vi "File check 2.0.vi"(8 "error in (no error)":errorcluster, 9 "reference":refnum<vi>, 10 "Numeric":i32, 11 "path":path) -> (0 "error out":errorcluster, 3 "Next State":string)   [LabVIEW 2016]
uses:
  Type Defs/File Check 2.0 control.ctl
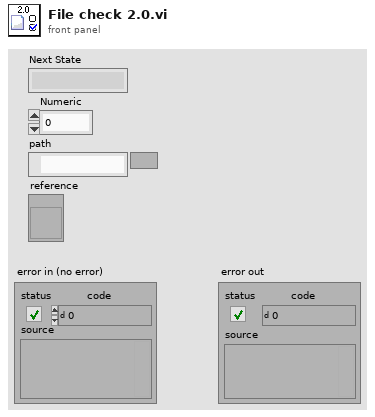
[diagram p1: front panel]
types:
  T1 = typedef "File Check 2.0 control.ctl" = enum16{"File Check", "Secondary check", "Refresh Google Drive"}
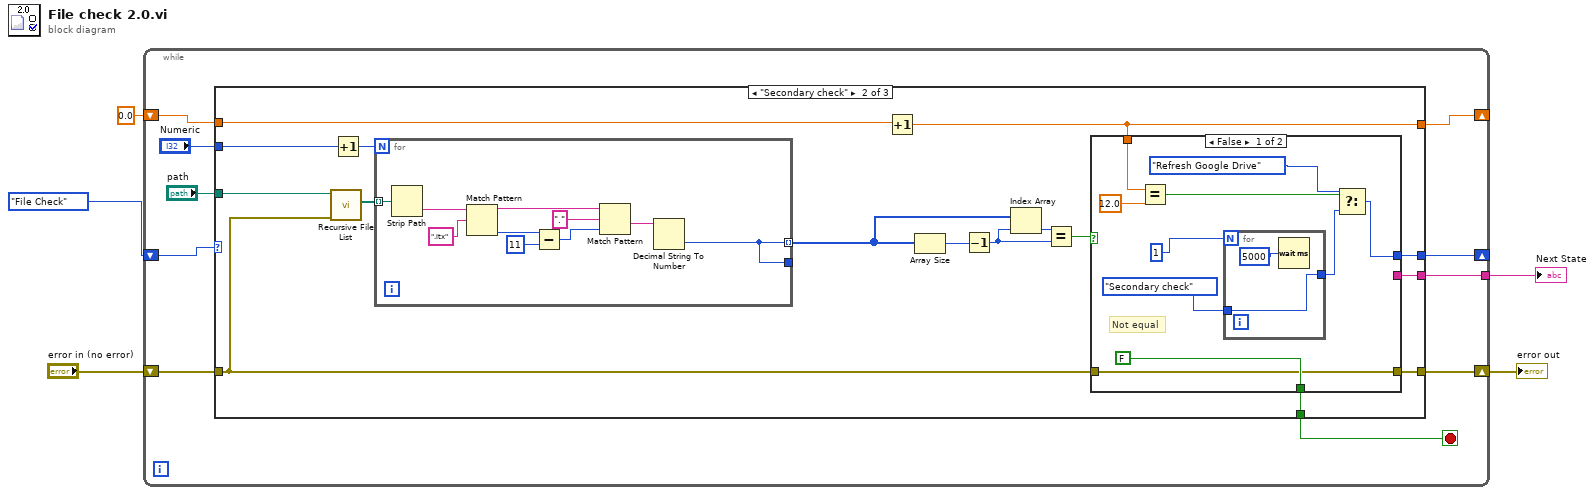
[diagram p0: block diagram]
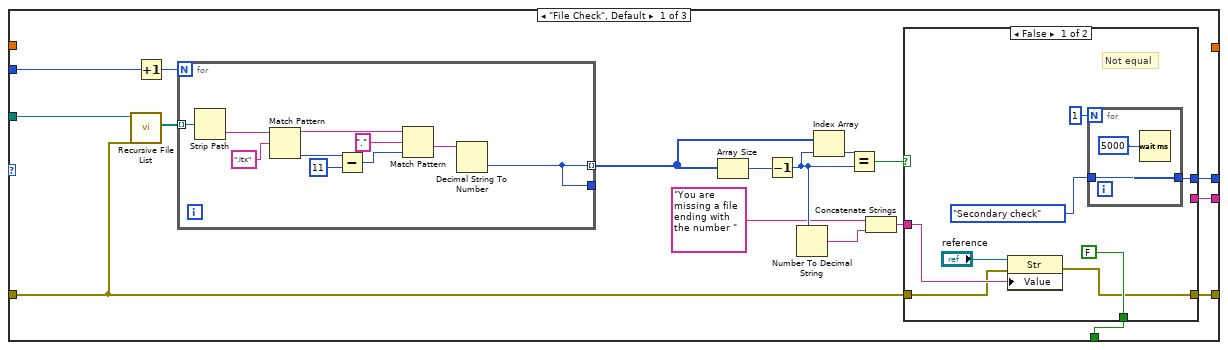
[diagram p2: hidden frame]
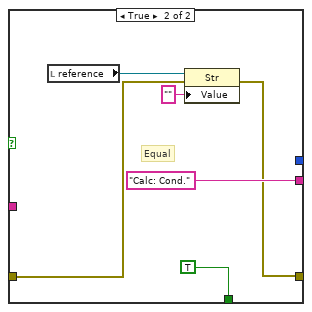
[diagram p3: hidden frame]
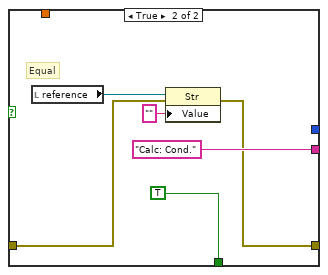
[diagram p4: hidden frame]
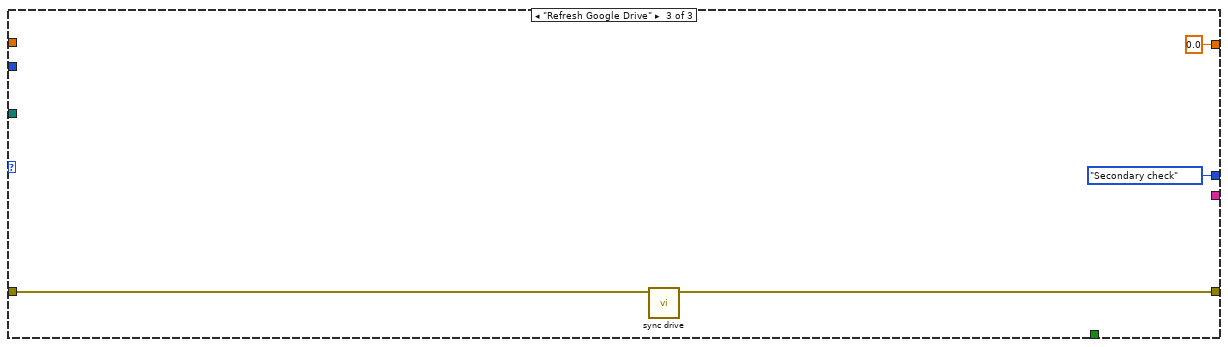
[diagram p5: hidden frame]
diagram:
  n1 = while {
    tunnel: [w15] -> w5
    shift-right: [w12] -> _
    shift-left: File_Check_2.0_control."File Check" -> [w11]
    shift-right: [w10] -> w2
    shift-left: "error in (no error)" -> [w7]
    shift-right: [w8] -> _
    shift-left: 0.0 -> [w9]
    stop <- w6 stop-if-true
    n2 = case shown="\"Secondary check\"" w11 {
      tunnel: [w25 w67 _] -> w15
      tunnel: [w23 w66 _] -> w6
      tunnel: "Numeric" -> [w26 w65 _]
      tunnel: "path" -> [w18 w63 _]
      tunnel: [w24 w64 File_Check_2.0_control."Secondary check"] -> w12
      tunnel: [w16 w62 w103] -> w10
      tunnel: w9 -> [_ w61 _]
      tunnel: [_ w60 0.0] -> w8
      tunnel: w7 -> [w17 w59 w104]
      frame "File Check", Default {
        n3 = call <vilib>:"Recursive File List.vi"("error in (no error)"=w17, "Folder Path"=w18) -> ("All Files in Dir"=w32:path[])  [unwired: 6 in, 3 out]
        n4 = Increment(x=w26) -> (x+1=w27:i32)
        n5 = for {
          N: w27 -> [_]
          tunnel: [w49] -> w28 mode=indexing
          tunnel: w32 -> [w50] mode=indexing
          tunnel: [w49] -> _
          n6 = Strip Path(path=w50) -> (name=w58:string)  [unwired: 1 out]
          n7 = Match Pattern(string=w58, regular expression=".itx") -> (before substring=w53:string, offset past match=w56:i32)  [unwired: 1 in, 2 out]
          n8 = Subtract(x=w56, y=11) -> (x-y=w54:i32)
          n9 = Match Pattern(string=w53, regular expression=".", offset (0)=w54) -> (after substring=w51:string)  [unwired: 3 out]
          n10 = Decimal String To Number(string=w51) -> (number=w49:i32)  [unwired: 2 in, 1 out]
        }
        n11 = Array Size(array=w28) -> (size(s)=w31:i32)
        n12 = Decrement(x=w31) -> (x-1=w22:i32)
        n13 = Number To Decimal String(number=w22) -> (decimal integer string=w20:string)  [unwired: 1 in]
        n14 = Index Array(array=w28, index=w22) -> (element=w30:i32)
        n15 = Equal?(x=w30, y=w22) -> (x = y?=w29:bool)
        n16 = Concatenate Strings("You are missing a file ending with the number " ("string"), w20) -> (w19:string)
        n17 = case shown="False" w29 {
          tunnel: [_ "Calc: Cond." ("Message")] -> w25
          tunnel: [FALSE TRUE] -> w23
          tunnel: [w39 _] -> w24
          tunnel: w19 -> [w35 _]
          tunnel: w17 -> [w34 w44]
          tunnel: [w33 w43] -> w16
          frame False {
            # "Not equal"
            n18 = property class="Str"(reference="reference", error in=w34, "Value"=w35) -> (error out=w33:errorcluster)  [unwired: 1 out]
            n19 = for {
              N: 1 -> [_]
              tunnel: [w41] -> w39
              tunnel: File_Check_2.0_control."Secondary check" -> [w41]
              n20 = Wait (ms)(milliseconds to wait=u32 5000) -> ()  [unwired: 1 out]
            }
          }
          frame True {
            # "Equal"
            n21 = local read "reference"() -> (w46:refnum<vi>)
            n22 = property class="Str"(reference=w46, error in=w44, "Value"="") -> (error out=w43:errorcluster)  [unwired: 1 out]
          }
        }
      }
      frame "Secondary check" {
        n23 = call <vilib>:"Recursive File List.vi"("error in (no error)"=w59, "Folder Path"=w63) -> ("All Files in Dir"=w74:path[])  [unwired: 6 in, 3 out]
        n24 = Increment(x=w65) -> (x+1=w68:i32)
        n25 = for {
          N: w68 -> [_]
          tunnel: [w93] -> w69 mode=indexing
          tunnel: w74 -> [w94] mode=indexing
          tunnel: [w93] -> _
          n26 = Strip Path(path=w94) -> (name=w102:string)  [unwired: 1 out]
          n27 = Match Pattern(string=w102, regular expression=".itx") -> (before substring=w97:string, offset past match=w100:i32)  [unwired: 1 in, 2 out]
          n28 = Subtract(x=w100, y=11) -> (x-y=w98:i32)
          n29 = Match Pattern(string=w97, regular expression=".", offset (0)=w98) -> (after substring=w95:string)  [unwired: 3 out]
          n30 = Decimal String To Number(string=w95) -> (number=w93:i32)  [unwired: 2 in, 1 out]
        }
        n31 = Increment(x=w61) -> (x+1=w60:dbl)
        n32 = Array Size(array=w69) -> (size(s)=w73:i32)
        n33 = Decrement(x=w73) -> (x-1=w70:i32)
        n34 = Index Array(array=w69, index=w70) -> (element=w72:i32)
        n35 = Equal?(x=w72, y=w70) -> (x = y?=w71:bool)
        n36 = case shown="False" w71 {
          tunnel: [_ "Calc: Cond." ("Message")] -> w67
          tunnel: [FALSE TRUE] -> w66
          tunnel: [w75 _] -> w64
          tunnel: w59 -> [w81 w88]
          tunnel: [w81 w87] -> w62
          tunnel: w60 -> [w79 _]
          frame False {
            # "Not equal"
            n37 = Equal?(x=w79, y=12.0) -> (x = y?=w76:bool)
            n38 = for {
              N: 1 -> [_]
              tunnel: File_Check_2.0_control."Secondary check" -> [w85]
              tunnel: [w85] -> w78
              n39 = Wait (ms)(milliseconds to wait=u32 5000) -> ()  [unwired: 1 out]
            }
            n40 = Select(t=File_Check_2.0_control."Refresh Google Drive", s=w76, f=w78) -> (s? t:f=w75:T1)
          }
          frame True {
            # "Equal"
            n41 = local read "reference"() -> (w90:refnum<vi>)
            n42 = property class="Str"(reference=w90, error in=w88, "Value"="") -> (error out=w87:errorcluster)  [unwired: 1 out]
          }
        }
      }
      frame "Refresh Google Drive" {
        n43 = call "sync drive.vi"("error in (no error)"=w104) -> ("error out"=w103:errorcluster)  [unwired: 10 in]
      }
    }
  }
  "Next State" <- w5
  "error out" <- w2
